vi "semafor_while_for.vi"() -> ()   [LabVIEW 2016]
panel:
  in  "Verde":i32
  in  "Galben":i32
  in  "Rosu":i32
  in  "stop":bool
  out "Verde":bool
  out "Galben":bool
  out "Rosu":bool
  out "Secunda":i32
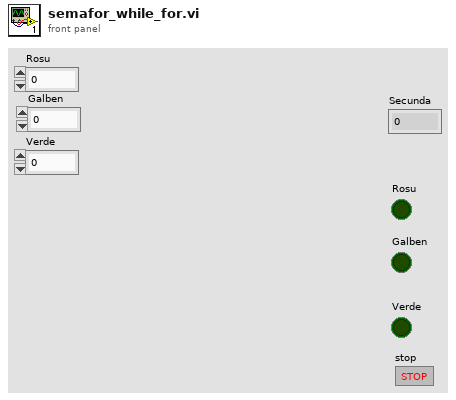
[diagram p1: front panel]
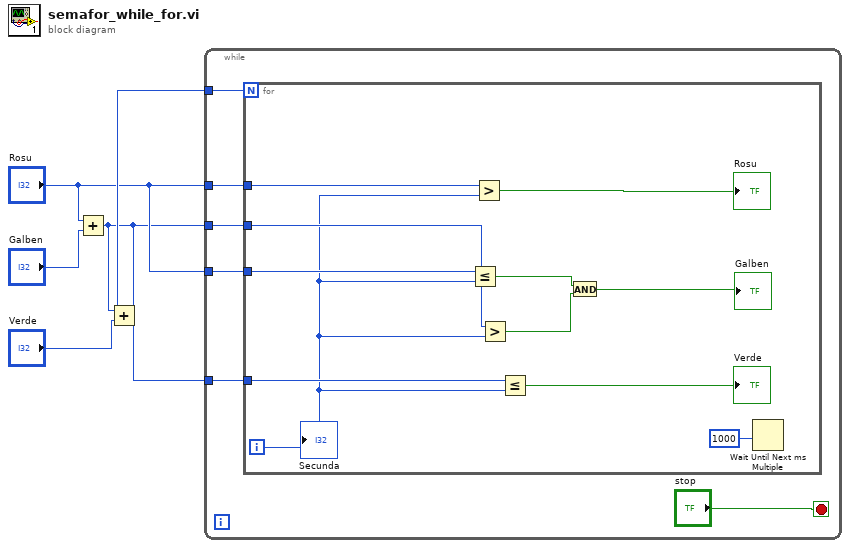
[diagram p0: block diagram]
diagram:
  n1 = Add(x="Rosu", y="Galben") -> (x+y=w1:i32)
  n2 = Add(x=w1, y="Verde") -> (x+y=w3:i32)
  n3 = while {
    tunnel: w3 -> [w11]
    tunnel: "Rosu" -> [w9]
    tunnel: "Rosu" -> [w8]
    tunnel: w1 -> [w7]
    tunnel: w1 -> [w6]
    stop <- "stop" stop-if-true
    n4 = for {
      N: w11 -> [_]
      tunnel: w9 -> [w21]
      tunnel: w8 -> [w19]
      tunnel: w7 -> [w18]
      tunnel: w6 -> [w14]
      i -> [w13]
      n5 = Less Or Equal?(x=w19, y=w13) -> (x <= y?=w17:bool)
      n6 = Greater?(x=w21, y=w13) -> (0:→"Rosu":bool)
      n7 = Greater?(x=w18, y=w13) -> (0:w16:bool)
      n8 = Less Or Equal?(x=w14, y=w13) -> (x <= y?=→"Verde":bool)
      n9 = And(x=w17, y=w16) -> (x .and. y?=→"Galben":bool)
      n10 = Wait Until Next ms Multiple(millisecond multiple=u32 1000) -> ()  [unwired: 1 out]
      "Secunda" <- w13
    }
  }
